vi "add set position(SubVI).vi"() -> (0 "布尔 3":bool, 2 "连接的字符串":string)   [LabVIEW 2019, in "SubVI.lvlib"]
uses:
  SubVI.lvlib
panel:
  in  "cancel":bool
  in  "ok":bool
  in  "Speed":i32 min=0 max=14
  in  "Position":dbl=2.0 min=0.0 max=400.0
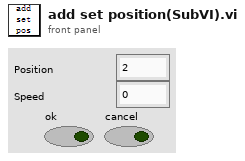
[diagram p1: front panel]
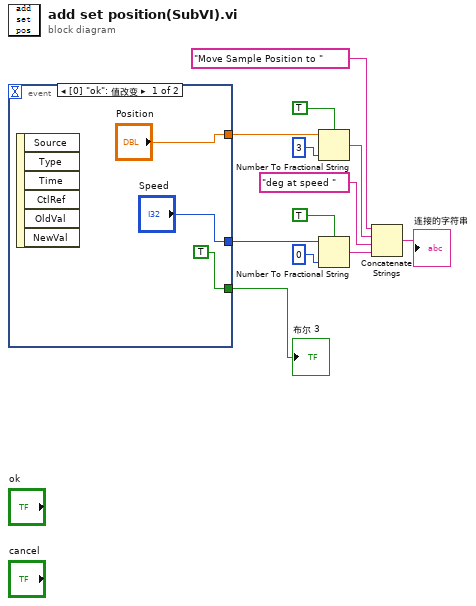
[diagram p0: block diagram]
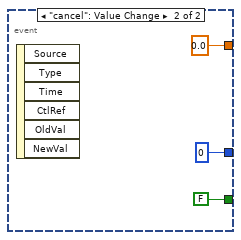
[diagram p2: hidden frame]
diagram:
  n1 = event shown="[0] \"ok\": 值改变" {
    selector: _ -> [_ _]
    dyn-events: _ -> [_ _]
    timeout: _ -> [_ _]
    tunnel: ["Speed" 0 ("Rate输入")] -> w3
    tunnel: ["Position" 0.0 ("Field")] -> w10
    tunnel: [TRUE FALSE] -> w12
    event "ok": Value Change {
      n2 = event-data() -> ()  [unwired: 1 in, 6 out]
    }
    event "cancel": Value Change {
      n3 = event-data() -> ()  [unwired: 1 in, 6 out]
    }
  }
  "布尔 3" <- w12
  n4 = Number To Fractional String(use system decimal point (T)=TRUE ("使用系统小数点(T)"), number=w10, precision (6)=i16 3 ("精度(6)")) -> (F-format string=w8:string)  [unwired: 1 in]
  n5 = Number To Fractional String(use system decimal point (T)=TRUE ("使用系统小数点(T)"), number=w3, precision (6)=i16 0 ("精度(6)")) -> (F-format string=w2:string)  [unwired: 1 in]
  n6 = Concatenate Strings("Move Sample Position to " ("字符串"), w8, "deg at speed " ("字符串"), w2) -> (→"连接的字符串":string)
